vi "Create Setpoint Trajectory.vi"() -> ()   [LabVIEW 2018]
uses:
  COBRA Iterative Learning Control Library.lvlib
panel:
  out "Phase":dbl[](graph)
  out "Position":dbl[](graph)
  out "XY Graph":cluster{"X":dbl, "Y":dbl}[](graph)
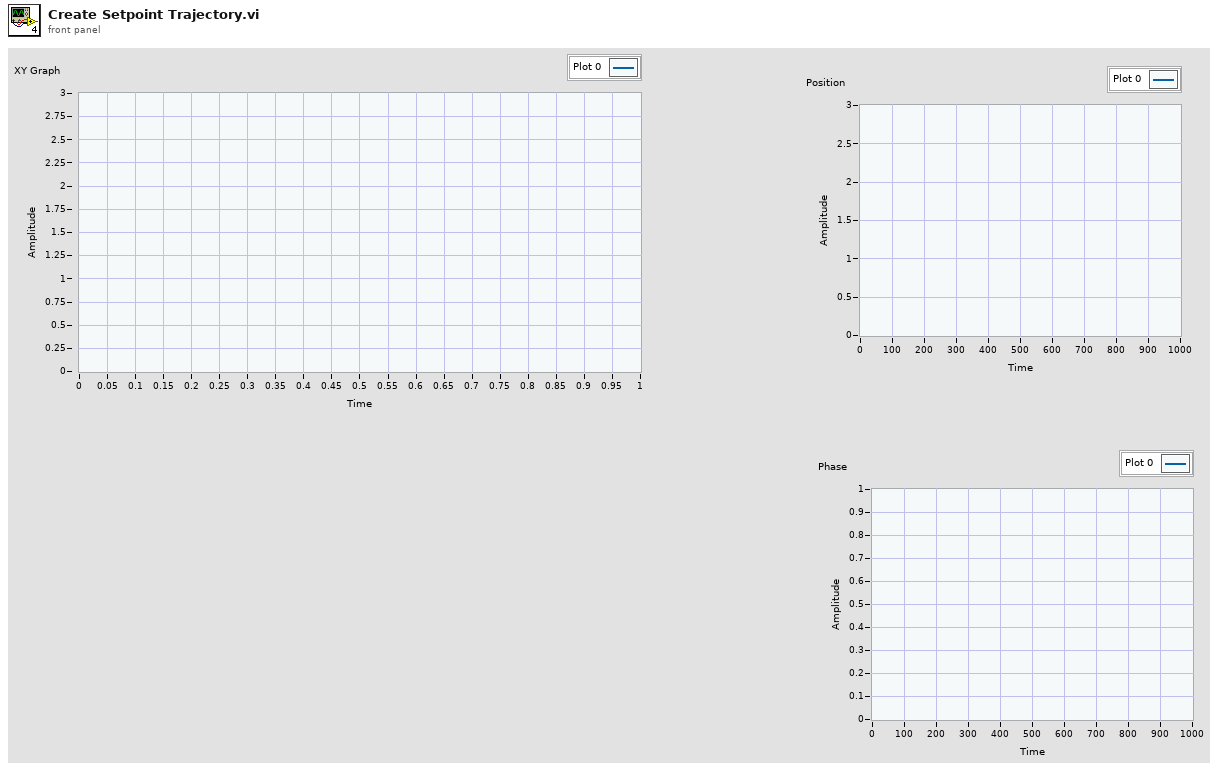
[diagram p1: front panel]
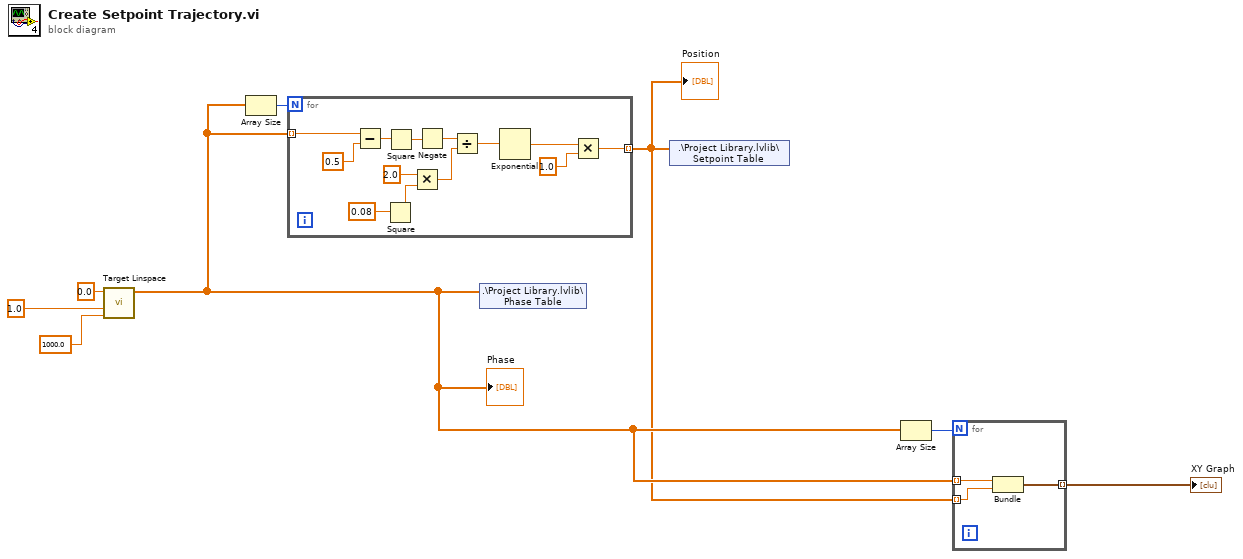
[diagram p0: block diagram]
diagram:
  n1 = call "Target Linspace.vi"("NumElements"=1000.0, "End"=1.0, "Start"=0.0) -> ("Array"=w2:dbl[])  [unwired: 8 in]
  "Phase" <- w2
  n2 = Array Size(array=w2) -> (size(s)=w5:i32)
  n3 = for {
    N: w5 -> [_]
    tunnel: w2 -> [w10] mode=indexing
    tunnel: [w9] -> w1 mode=indexing
    n4 = Subtract(x=w10, y=0.5) -> (x-y=w20:dbl)
    n5 = Square(x=0.08 ("y")) -> (x^2=w15:dbl)
    n6 = Square(x=w20) -> (x^2=w19:dbl)
    n7 = Multiply(x=2.0, y=w15) -> (x*y=w14:dbl)
    n8 = Negate(x=w19) -> (-x=w18:dbl)
    n9 = Divide(x=w18, y=w14) -> (x/y=w13:dbl)
    n10 = Exponential(1:w13) -> (0:w12:dbl)
    n11 = Multiply(x=w12, y=1.0) -> (x*y=w9:dbl)
  }
  "Position" <- w1
  n12 = shared-variable ".\\Project Library.lvlib\\Phase Table"(w2) -> ()  [unwired: 1 in, 1 out]
  n13 = shared-variable ".\\Project Library.lvlib\\Setpoint Table"(w1) -> ()  [unwired: 1 in, 1 out]
  n14 = Array Size(array=w2) -> (size(s)=w4:i32)
  n15 = for {
    N: w4 -> [_]
    tunnel: w2 -> [w24] mode=indexing
    tunnel: w1 -> [w23] mode=indexing
    tunnel: [w22] -> w3 mode=indexing
    n16 = Bundle("Numeric"=w24, w23) -> (w22:cluster{"Numeric":dbl, dbl})  [unwired: 1 in]
  }
  "XY Graph" <- w3
